vi "Write To tmp Directory.vi"(7 "operation (0:open)":T1(ring)=enum."replace or create", 8 "error in (no error)":errorcluster, 10 "sketch name":string="out", 11 "arduino code":string="/*  Program generated by SimpleArduinoTranscriptor\nby LuboJ.\n*/\nvoid setup(){\nSerial.begin(9600); \n}\nvoid loop(){\ndelay(50);\nSerial.println(\"Hello world!\"); \n}\n") -> (0 "error out":errorcluster={"status"=TRUE, "code"=10, "source"="Create Folder in Write To tmp Directory.vi->Test Simple Arduino Program 1.vi<APPEND>\nC:\\Users\\lubo\\Documents\\LabView\\Simple-Arduino-Transcriptor\\tmp\\out"}, 3 "output file":path=path "C:/Users/lubo/Documents/LabView/Simple-Arduino-Transcriptor/tmp/out/out.ino")   [LabVIEW 2014]
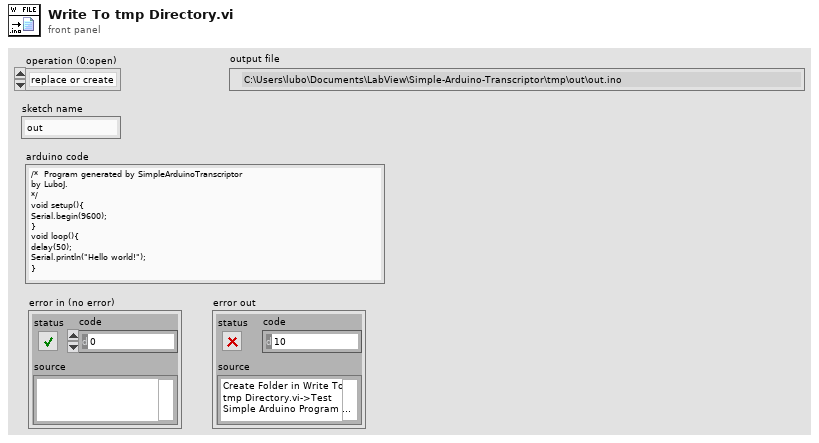
[diagram p1: front panel]
types:
  T1 = enum16{"open", "replace", "create", "open or create", "replace or create", "replace or create with confirmation"}
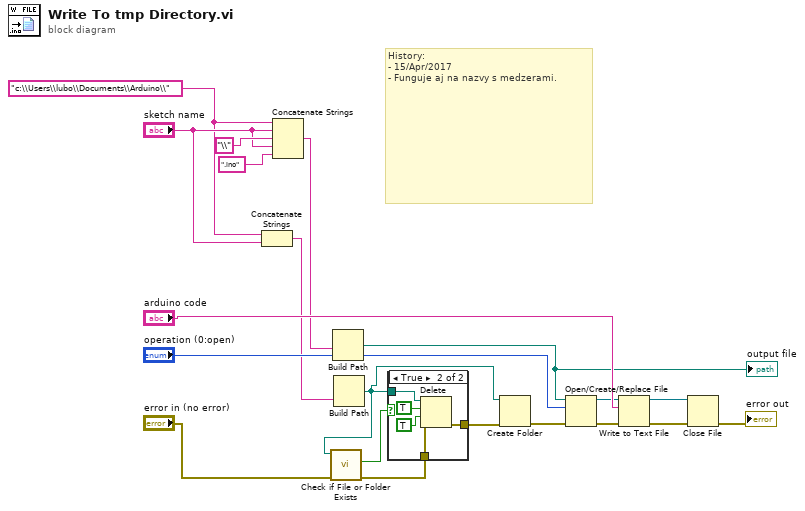
[diagram p0: block diagram]
diagram:
  w1 = "c:\\Users\\lubo\\Documents\\Arduino\\" ("name or relative path")
  # "History:\n- 15/Apr/2017\n- Funguje aj na nazvy s medzerami."
  n1 = Concatenate Strings(w1, "sketch name") -> (w7:string)
  n2 = Concatenate Strings(w1, "sketch name", "\\" ("string"), "sketch name", ".ino" ("string")) -> (w13:string)
  n3 = Build Path(name or relative path=w13) -> (appended path=w12:path)  [unwired: 1 in]
  "output file" <- w12
  n4 = Build Path(name or relative path=w7) -> (appended path=w2:path)  [unwired: 1 in]
  n5 = call <vilib>:"Check if File or Folder Exists.vi"("error in (no error)"="error in (no error)", "path"=w2) -> ("error out"=w5:errorcluster, "file or folder exists?"=w4:bool)  [unwired: 7 in, 1 out]
  n6 = case shown="True" w4 {
    tunnel: w2 -> [_ w25]
    tunnel: w5 -> [w21 w23]
    tunnel: [w21 w22] -> w3
    frame False {
    }
    frame True {
      n7 = Delete(path (use dialog)=w25, entire hierarchy (F)=TRUE, confirm (F)=TRUE, error in=w23) -> (error out=w22:errorcluster)  [unwired: 1 in, 2 out]
    }
  }
  n8 = Create Folder(path (use dialog)=w2, error in=w3) -> (error out=w9:errorcluster)  [unwired: 1 in, 2 out]
  n9 = Open/Create/Replace File(file path (use dialog)=w12, error in=w9, operation (0:open)="operation (0:open)") -> (refnum out=w16:refnum<file>, error out=w15:errorcluster)  [unwired: 3 in, 1 out]
  n10 = Write to Text File(file (use dialog)=w16, text="arduino code", error in=w15) -> (refnum out=w20:refnum<file>, error out=w18:errorcluster)  [unwired: 1 in, 1 out]
  n11 = Close File(refnum=w20, error in=w18) -> (error out=→"error out":errorcluster)  [unwired: 1 out]
